vi "Check CTRL Coordinates.vi"(9 "Object Coords Array In":T2[](array[typedef]), 11 "Mouse Coords In":T1) -> (3 "Index Out":i32)   [LabVIEW 2012]
uses:
  <vilib>/Utility/miscctls.llb/LVRectTypeDef.ctl
  <vilib>/Utility/miscctls.llb/LVPoint32TypeDef.ctl
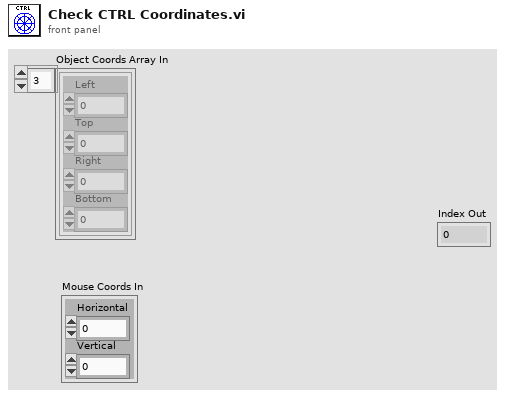
[diagram p1: front panel]
types:
  T1 = typedef "LVPoint32TypeDef.ctl" = cluster{"Horizontal":i32, "Vertical":i32}
  T2 = typedef "LVRectTypeDef.ctl" = cluster{"Left":i16, "Top":i16, "Right":i16, "Bottom":i16}
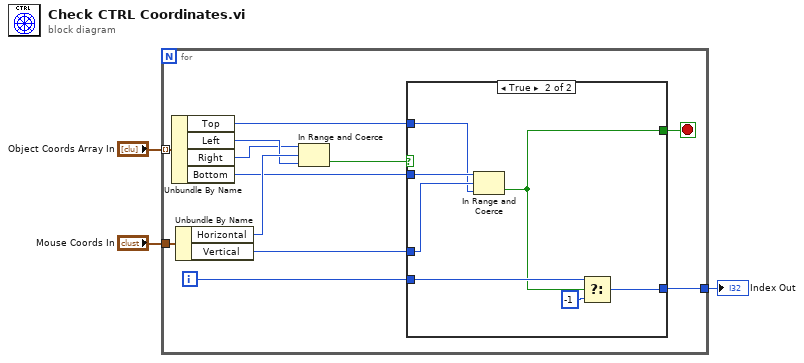
[diagram p0: block diagram]
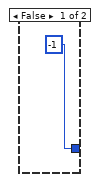
[diagram p2: hidden frame]
diagram:
  n1 = for {
    tunnel: "Object Coords Array In" -> [w15] mode=indexing
    tunnel: "Mouse Coords In" -> [w14]
    tunnel: [w10] -> w1
    i -> [w13]
    stop <- w9 stop-if-true
    n2 = Unbundle By Name(w15) -> ("Top"=w12:i16, "Left"=w7:i16, "Right"=w5:i16, "Bottom"=w4:i16)
    n3 = Unbundle By Name(w14) -> ("Horizontal"=w8:i32, "Vertical"=w11:i32)
    n4 = In Range and Coerce(upper limit=w5, x=w8, lower limit=w7) -> (In Range?=w6:bool)  [unwired: 1 out]
    n5 = case shown="True" w6 {
      tunnel: w13 -> [_ w23]
      tunnel: w12 -> [_ w17]
      tunnel: w11 -> [_ w19]
      tunnel: [-1 ("f") w21] -> w10
      tunnel: [_ w20] -> w9
      tunnel: w4 -> [_ w18]
      frame False {
      }
      frame True {
        n6 = In Range and Coerce(upper limit=w18, x=w19, lower limit=w17) -> (In Range?=w20:bool)  [unwired: 1 out]
        n7 = Select(t=w23, s=w20, f=-1) -> (s? t:f=w21:i32)
      }
    }
  }
  "Index Out" <- w1
